vi "生产异常统计.vi"(11 "data输入":string[](array[string])) -> (0 "tablename":string, 3 "data":string[](array[string]))   [LabVIEW 2017]
uses:
  Sqlite/CBB/ReadAllData.vi
  Sqlite/SQLite.lvlib
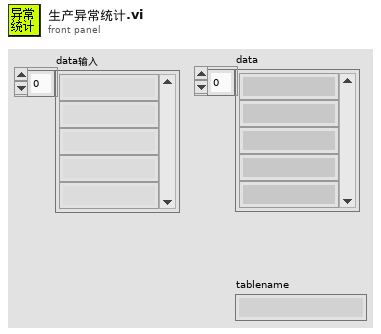
[diagram p1: front panel]
types:
  T1 = typedef "pathcheck选项.ctl" = enum16{"ProductData", "CTData", "ERData", "IOTDATA"}
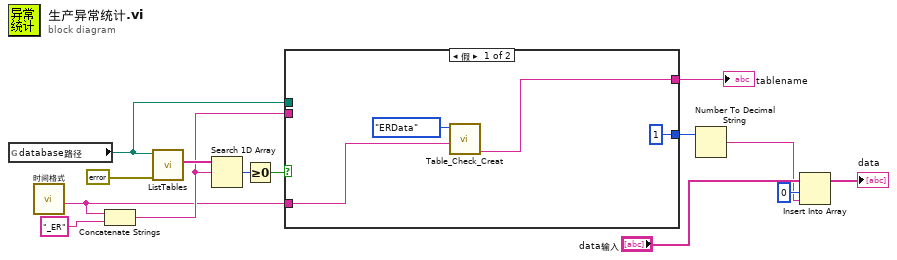
[diagram p0: block diagram]
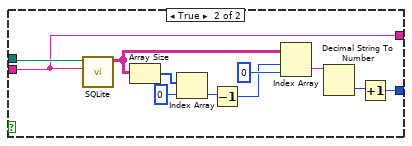
[diagram p2: hidden frame]
diagram:
  n1 = global read "数据库全局.vi" "database路径"() -> (w9:path)
  n2 = call "时间格式.vi"() -> ("_Date"=w7:string)  [unwired: 7 in, 4 out]
  n3 = Concatenate Strings(w7, "_ER" ("字符串")) -> (w8:string)
  n4 = call "ListTables.vi"("error in (no error)"=errorcluster {"status"=FALSE, "code"=0, "source"=""}, "DbPath"=w9) -> ("Tables"=w13:string[])  [unwired: 6 in, 3 out]
  n5 = Search 1D Array(1D array=w13, element=w8) -> (index of element=w14:i32)  [unwired: 1 in]
  n6 = Greater Or Equal To 0?(x=w14) -> (x >= 0?=w10:bool)
  n7 = case shown="假" w10 {
    tunnel: w9 -> [_ w29]
    tunnel: w8 -> [_ w19]
    tunnel: [1 w20] -> w5
    tunnel: w7 -> [w16 _]
    tunnel: [w15 w19] -> w6
    frame False {
      n8 = call "Table_Check_Creat.vi"("_datetime"=w16, "pathcheck选项"=pathcheck选项."ERData") -> ("tablename"=w15:string)  [unwired: 7 in, 2 out]
    }
    frame True {
      n9 = call-poly "SQLite.vi"("Table Name"=w19, "DbPath"=w29) -> ("Results"=w27:string[][])  [unwired: 4 in, 5 out]
      n10 = Array Size(array=w27) -> (size(s)=w26:i32[])
      n11 = Index Array(array=w26, index=0 ("索引")) -> (element=w24:i32)
      n12 = Decrement(x=w24) -> (x-1=w23:i32)
      n13 = Index Array(array=w27, index (row)=w23, index (col)=0 ("禁用的索引 (列)")) -> (element=w22:string)
      n14 = Decimal String To Number(string=w22) -> (number=w21:i32)  [unwired: 2 in, 1 out]
      n15 = Increment(x=w21) -> (x+1=w20:i32)
    }
  }
  "tablename" <- w6
  n16 = Number To Decimal String(number=w5) -> (decimal integer string=w2:string)  [unwired: 1 in]
  n17 = Insert Into Array(array="data输入", index=0 ("索引"), new element=w2) -> (→"data":string[])
